vi "TEST_LoadObserverControlMatrix_singleAxis_linear.vi"() -> ()   [LabVIEW 2017]
uses:
  typeDefs/Bz_bram.ctl
  typeDefs/Lz_bram.ctl
  typeDefs/Kz_bram.ctl
  typeDefs/A_as_vec_bram.ctl
  typeDefs/Nx_bram.ctl
  <vilib>/rvi/Emulation/niFpgaGetClockAttributes.vi
  <vilib>/rvi/Emulation/niFpgaSctlEmulationGetInTimedLoop.vi
  <vilib>/rvi/Emulation/niFpgaEmulationReportErrorSimple.vi
  <vilib>/rvi/Emulation/niFpgaCriticalErrorInLSC.vi
panel:
  in  "Mem Select":T1(ring)=enum."L_col1"
  out "Array":fxp<+/-,32,3>[](array[numeric])
  in  "stop":bool
  in  "Row start":u16
  in  "Ns":u16
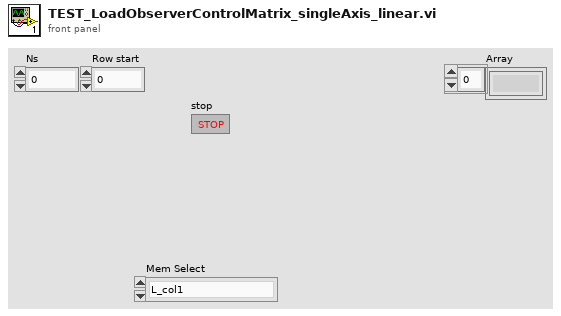
[diagram p1: front panel]
types:
  T1 = enum16{"Bz_col1", "L_col1", "K_row1", "Az", "Nx_col1", ""}
  T2 = typedef "Bz_bram.ctl" = refnum<k21>
  T3 = typedef "Lz_bram.ctl" = refnum<k21>
  T4 = typedef "Kz_bram.ctl" = refnum<k21>
  T5 = typedef "A_as_vec_bram.ctl" = refnum<k21>
  T6 = typedef "Nx_bram.ctl" = refnum<k21>
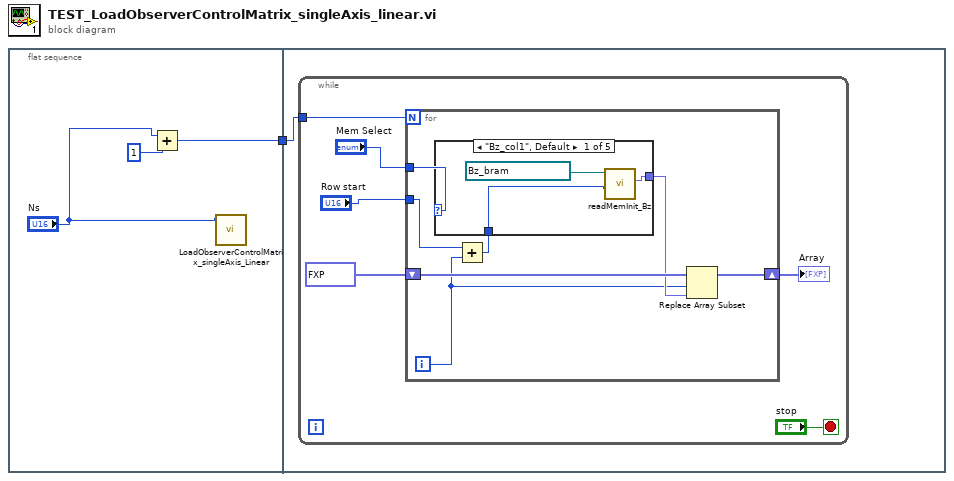
[diagram p0: block diagram]
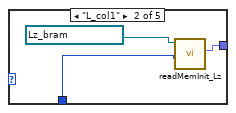
[diagram p2: hidden frame]
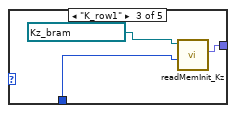
[diagram p3: hidden frame]
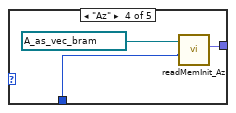
[diagram p4: hidden frame]
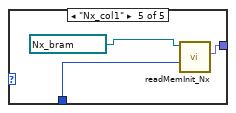
[diagram p5: hidden frame]
diagram:
  n1 = flat-sequence {
    tunnel: [w3] -> w1
    tunnel: w1 -> [w5]
    frame #0 {
      n2 = Add(x="Ns", y=u16 1) -> (x+y=w3:u16)
      n3 = call "LoadObserverControlMatrix_singleAxis_Linear.vi"("NS_obs/cntrl"="Ns") -> ()  [unwired: 10 in, 1 out]
    }
    frame #1 {
      n4 = while {
        tunnel: w5 -> [w11]
        stop <- "stop" stop-if-true
        n5 = for {
          N: w11 -> [_]
          tunnel: "Mem Select" -> [w15]
          shift-right: [w17] -> w8
          shift-left: fxp<+/-,32,3>[] [0.0, 0.0, 0.0, 0.0, 0.0, 0.0, 0.0, 0.0, 0.0, 0.0, 0.0, 0.0, 0.0, 0.0, 0.0, 0.0, 0.0, 0.0, 0.0, 0.0, 0.0, 0.0, 0.0, 0.0, 0.0, 0.0, 0.0, 0.0, 0.0, 0.0, 0.0, 0.0, 0.0, 0.0, 0.0, 0.0, 0.0, 0.0, 0.0, 0.0, 0.0, 0.0, 0.0, 0.0, 0.0, 0.0, 0.0, 0.0, 0.0, 0.0] -> [w18]
          tunnel: "Row start" -> [w12]
          i -> [w13]
          n6 = Add(x=w12, y=w13) -> (x+y=w14:i32)
          n7 = case shown="\"Bz_col1\", Default" w15 {
            tunnel: w14 -> [w20 w23 w27 w29 w32]
            tunnel: [w21 w24 w26 w30 w33] -> w16
            frame "Bz_col1", Default {
              n8 = call "readMemInit_Bz.vi"("address"=w20, "Bz"=T2 "Bz_FXP_col1" ("Memory")) -> ("Data"=w21:fxp<+/-,32,2>)  [unwired: 9 in]
            }
            frame "L_col1" {
              n9 = call "readMemInit_Lz.vi"("address"=w23, "Lz"=T3 "L_FXP_col1" ("Memory")) -> ("Data"=w24:fxp<+/-,32,2>)  [unwired: 9 in]
            }
            frame "K_row1" {
              n10 = call "readMemInit_Kz.vi"("address"=w27, "Kz"=T4 "K_FXP_row1" ("Memory")) -> ("Data"=w26:fxp<+/-,32,2>)  [unwired: 9 in]
            }
            frame "Az" {
              n11 = call "readMemInit_Az.vi"("address"=w29, "Az_vec"=T5 "AasCol _FXP" ("Memory In")) -> ("Data"=w30:fxp<+/-,32,2>)  [unwired: 9 in]
            }
            frame "Nx_col1" {
              n12 = call "readMemInit_Nx.vi"("address"=w32, "Nx"=T6 "Nx_col1") -> ("Data"=w33:fxp<+/-,32,2>)  [unwired: 9 in]
            }
          }
          n13 = Replace Array Subset(array=w18, new element=w16, index=w13) -> (w17:fxp<+/-,32,3>[])
        }
        "Array" <- w8
      }
    }
  }
